vi "Get Supported Mode 1 PIDs.vi"(8 "error in (no error)":errorcluster, 10 "Cluster":cluster{i32[], i32[], i32[]}, 11 "VISA Refnum in":refnum<visa-resource-name>) -> (0 "error out":errorcluster, 1 "Supported PIDs":u32[](array[numeric]), 3 "Array":string[](array[string]))   [LabVIEW 2011]
uses:
  PID/Supported PIDs/Supported PIDs Folder/Supported PIDs.lvclass
  PID/PID.lvclass
panel:
  out "Array 2":i32[][](array[numeric])
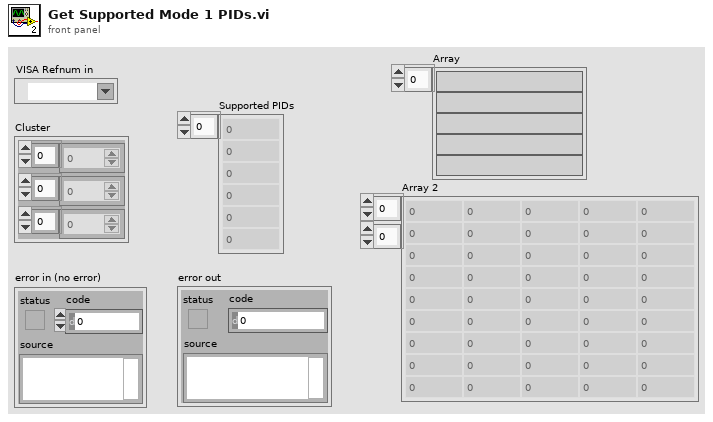
[diagram p1: front panel]
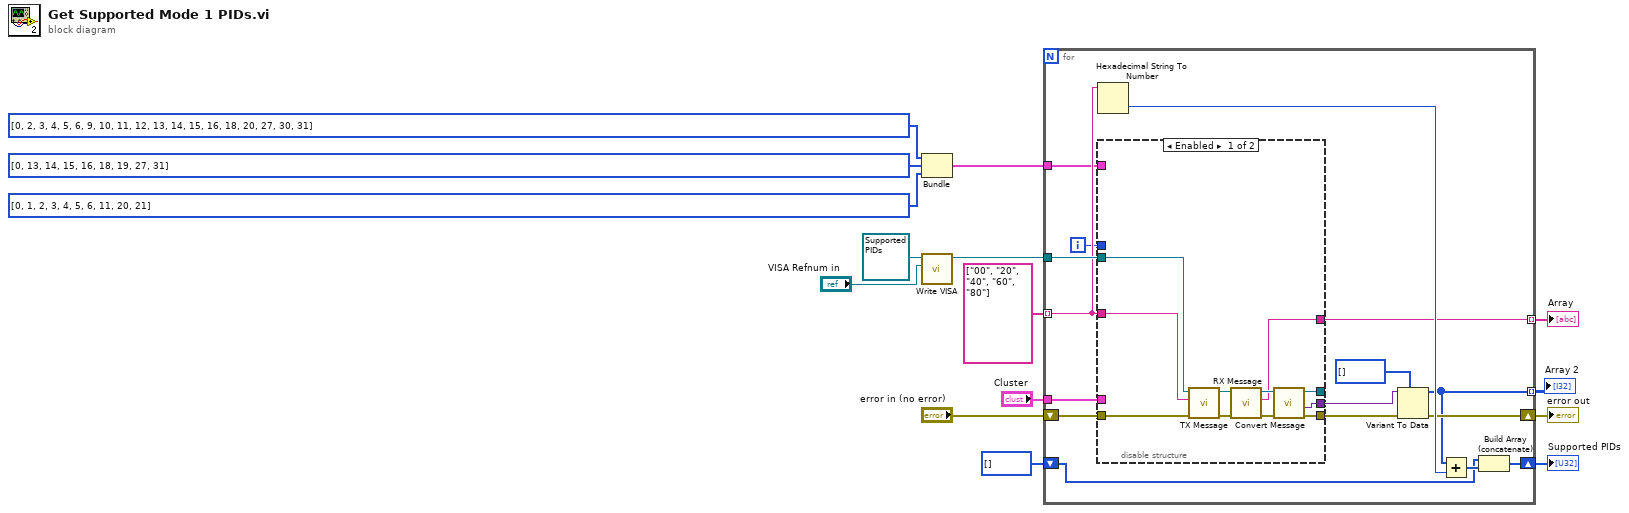
[diagram p0: block diagram]
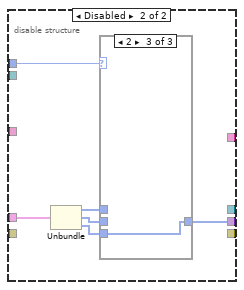
[diagram p2: hidden frame]
diagram:
  n1 = Bundle(i32[] [0, 2, 3, 4, 5, 6, 9, 10, 11, 12, 13, 14, 15, 16, 18, 20, 27, 30, 31], i32[] [0, 13, 14, 15, 16, 18, 19, 27, 31], i32[] [0, 1, 2, 3, 4, 5, 6, 11, 20, 21]) -> (w2:cluster{i32[], i32[], i32[]})  [unwired: 1 in]
  n2 = call "Write VISA.vi"("VISA"="VISA Refnum in", "PID in"=refnum<class "Supported PIDs.lvclass"> refnum ("Supported PIDs.lvclass")) -> ("PID out"=w9:refnum<class "Supported PIDs.lvclass">)  [unwired: 8 in, 1 out]
  n3 = for {
    tunnel: w9 -> [w31]
    tunnel: string[] ["00", "20", "40", "60", "80"] -> [w25] mode=indexing
    shift-right: [w27] -> w13
    shift-left: u32[] [] -> [w26]
    shift-right: [w21] -> w11
    shift-left: "error in (no error)" -> [w23]
    tunnel: w2 -> [w20]
    tunnel: "Cluster" -> [w19]
    tunnel: [w17] -> w15 mode=indexing
    tunnel: [w16] -> w1 mode=indexing
    i -> [w18]
    n4 = Hexadecimal String To Number(string=w25) -> (number=w24:u32)  [unwired: 2 in, 1 out]
    n5 = disable-structure shown="Enabled" {
      disable-tunnel: w31 -> [w40 _]
      disable-tunnel: [w37 w46] -> w30
      disable-tunnel: w25 -> [w36 _]
      disable-tunnel: w23 -> [w35 _]
      disable-tunnel: [w34 _] -> w22
      disable-tunnel: w20 -> [_ _]
      disable-tunnel: w19 -> [_ w48]
      disable-tunnel: w18 -> [_ w47]
      disable-tunnel: [w33 _] -> _
      disable-tunnel: [w32 _] -> w17
      frame Enabled {
        n6 = call-dynamic "TX Message.vi"("error in (no error)"=w35, "variant"=w36, "Engine RPM in"=w40) -> ("error out"=w38:errorcluster, "Engine RPM out"=w41:refnum<class "Supported PIDs.lvclass">)  [unwired: 7 in]
        n7 = call-dynamic "RX Message.vi"("error in (no error)"=w38, "PID in"=w41) -> ("error out"=w39:errorcluster, "String"=w32:string, "PID out"=w42:refnum<class "Supported PIDs.lvclass">)  [unwired: 7 in]
        n8 = call-dynamic "Convert Message.vi"("error in (no error)"=w39, "Supporting PIDs in"=w42) -> ("error out"=w34:errorcluster, "variant"=w37:variant, "Supporting PIDs out"=w33:refnum<class "Supported PIDs.lvclass">)  [unwired: 6 in, 1 out]
      }
      frame Disabled {
        n9 = Unbundle(w48) -> (w45:i32[], w44:i32[], w43:i32[])
        n10 = case shown="2" w47 {
          tunnel: [w49 w50 w51] -> w46
          tunnel: w45 -> [w49 _ _]
          tunnel: w44 -> [_ w50 _]
          tunnel: w43 -> [_ _ w51]
          frame 0, Default {
          }
          frame 1 {
          }
          frame 2 {
          }
        }
      }
    }
    n11 = Variant To Data(error in=w22, type=i32[] [], Variant=w30) -> (data=w16:i32[], error out=w21:errorcluster)
    n12 = Add(x=w16, y=w24) -> (x+y=w28:u32[])
    n13 = Build Array (concatenate)(w26, w28) -> (w27:u32[])
  }
  "Array" <- w15
  "Supported PIDs" <- w13
  "error out" <- w11
  "Array 2" <- w1
